vi "Initialize.vi"(8 "Error In":errorcluster) -> (0 "Error Out":errorcluster)   [LabVIEW 2015, in "Logger.lvlib"]
uses:
  Logger.lvlib
  Private/_Logger Action.ctl
  Private/File/_Action.ctl
  Private/_Control Action.ctl
  Private/Error/_Action.ctl
  Private/File/File.lvlib
  Private/Error/Error.lvlib
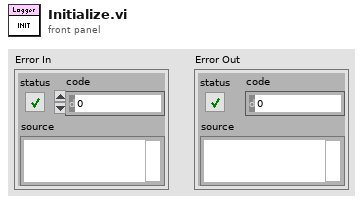
[diagram p1: front panel]
types:
  T1 = typedef "Logger.lvlib/Error.lvlib/_Action.ctl" = enum16{"Initialize", "Get", "Set Verbosity", "Set User-Defined Codes", "Set User-Defined Descriptions", "Shutdown"}
  T2 = typedef "Logger.lvlib/_Control Action.ctl" = enum16{"Initialize", "Get", "Set", "Shutdown"}
  T3 = typedef "Logger.lvlib/File.lvlib/_Action.ctl" = enum16{"Initialize", "Set Maximum File Size", "Set Maximum File Count", "Set Root Folder", "Set Enable Calendar Folder Tree", "Set File Extension", "Start", "Write", "Stop", "Shutdown"}
  T4 = typedef "Logger.lvlib/_Logger Action.ctl" = enum16{"Initialize", "Register", "Log", "Unregister", "Set Level", "Shutdown"}
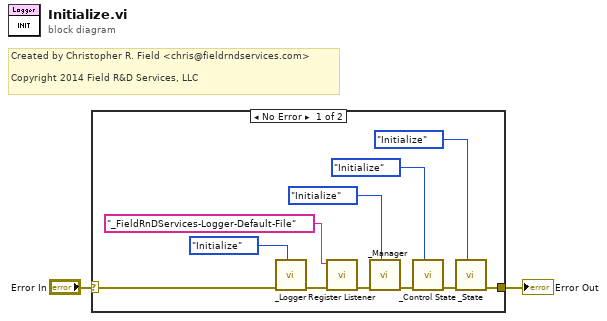
[diagram p0: block diagram]
diagram:
  # "Created by Christopher R. Field <chris@fieldrndservices.com>\n\nCopyright 2014 Field R&D Services, LLC"
  n1 = case shown="No Error" "Error In" {
    selector: "Error In" -> [w12 w14]
    tunnel: [w4 w14] -> w1
    frame No Error {
      n2 = call "_Logger.vi"("Action"=_Logger_Action."Initialize", "Error In"=w12) -> ("Error Out"=w11:errorcluster)  [unwired: 9 in]
      n3 = call "Register Listener.vi"("Error In"=w11, "Listener ID"="_FieldRnDServices-Logger-Default-File") -> ("Error Out"=w5:errorcluster)  [unwired: 9 in]
      n4 = call "_Manager.vi"("Action"=_Action."Initialize", "Error In"=w5) -> ("Error Out"=w9:errorcluster)  [unwired: 9 in]
      n5 = call "_Control State.vi"("Action"=_Control_Action."Initialize", "Error In"=w9) -> ("Error Out"=w7:errorcluster)  [unwired: 8 in, 1 out]
      n6 = call "_State.vi"("Action"=_Action."Initialize", "Error In"=w7) -> ("Error Out"=w4:errorcluster)  [unwired: 8 in, 1 out]
    }
    frame Error {
    }
  }
  "Error Out" <- w1
